vi "carPark.vi"() -> ()   [LabVIEW 2022 SP3]
doc: "This example demonstrates how you can use fuzzy logic to park a vehicle in a specified location."
uses:
  <vilib>/addons/Fuzzy Logic/FL Fuzzy Controller (MISO).vi
  <vilib>/addons/Fuzzy Logic/NI_Fuzzy_Logic_API.lvlib
panel:
  in  "Manual / Fuzzy":bool
  out "Steering Angle":picture
  out "Arrived":bool
  out "Steering Wheel":dbl
  in  "Initial Vehicle Angle":dbl(knob)=-56.0 min=-90.0 max=270.0 step=1.0 scale=-90.0..270.0
  in  "Stop":bool
  out "Grid":cluster{dbl[], dbl[]}[](graph)
  out "Car parking":picture
  # "Garage"
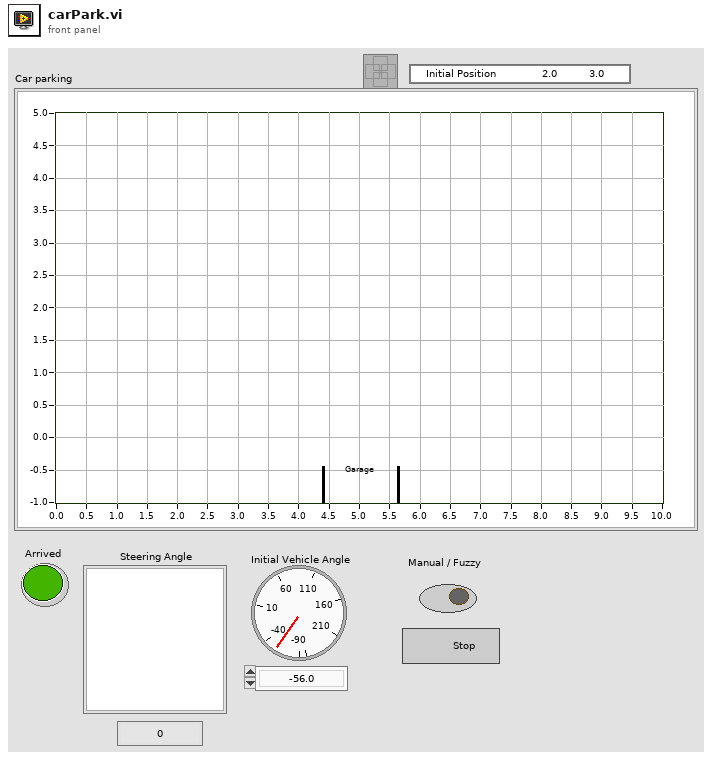
[diagram p1: front panel]
types:
  T1 = typedef "NI_Fuzzy_Logic_API.lvlib/FL System.ctl" = cluster{"input variables":T2[], "output variables":T2[], "rules":T5[], "defuzzification method":T11, "description":string, "user MF interpolating polynomials":T12[]}
  T2 = typedef "NI_Fuzzy_Logic_API.lvlib/FL Variable.ctl" = cluster{"name":string, "range":dbl[], "MFs":T3[]}
  T3 = typedef "NI_Fuzzy_Logic_API.lvlib/FL Membership Function.ctl" = cluster{"name":string, "shape":T4, "points":dbl[], "color":u32, "user-defined shape index":i32}
  T4 = typedef "NI_Fuzzy_Logic_API.lvlib/FL Membership Function Shape.ctl" = u16
  T5 = typedef "NI_Fuzzy_Logic_API.lvlib/FL Rule.ctl" = cluster{"antecedents":T6[], "antecedent connective":T8, "consequents":T9[], "consequent implication":T10, "degree of support":dbl}
  T6 = typedef "NI_Fuzzy_Logic_API.lvlib/FL Antecedent.ctl" = cluster{"Var Index":i32, "MF Index":i32, "Cond":T7}
  T7 = typedef "NI_Fuzzy_Logic_API.lvlib/FL Modifier.ctl" = u16
  T8 = typedef "NI_Fuzzy_Logic_API.lvlib/FL Antecedent Connective.ctl" = u16
  T9 = typedef "NI_Fuzzy_Logic_API.lvlib/FL Consequent.ctl" = cluster{"Var Index":i32, "MF Index":i32, "Cond":T7}
  T10 = typedef "NI_Fuzzy_Logic_API.lvlib/FL Consequent Implication.ctl" = u16
  T11 = typedef "NI_Fuzzy_Logic_API.lvlib/FL Defuzzification.ctl" = u16
  T12 = typedef "NI_Fuzzy_Logic_API.lvlib/FL Interpolating polynomials.ctl" = cluster{"X":dbl[], "Y":dbl[], "Y(x) coeff":dbl[][], "X(y) coeff":dbl[][], "Area(y) coeff":dbl[][], "coa_x(y) coeff":dbl[][]}
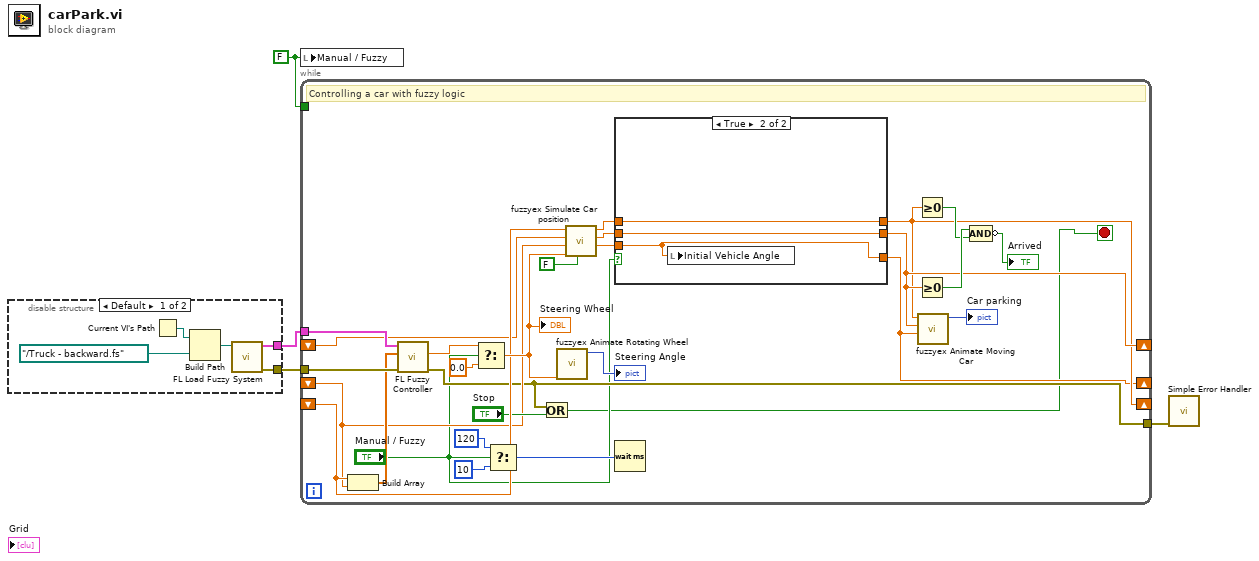
[diagram p0: block diagram]
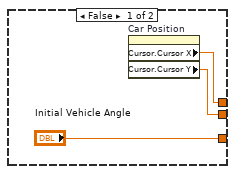
[diagram p3: hidden frame]
diagram:
  w2 = FALSE ("Operation Mode")
  n1 = disable-structure shown="Default" {
    disable-tunnel: [w7 _] -> w4
    disable-tunnel: [w6 _] -> w3
    frame condition #0 (active) {
      n2 = Current VI's Path() -> (path=w5:path)
      n3 = Build Path(base path=w5, name or relative path=path "../Truck - backward.fs") -> (appended path=w9:path)
      n4 = call <vilib>:"FL Load Fuzzy System.vi"("file path"=w9) -> ("error out"=w7:errorcluster, "fuzzy system out"=w6:T1)  [unwired: 1 in, 8 out]
    }
    frame condition #1 {
    }
  }
  n5 = local write "Manual / Fuzzy"(w2) -> ()
  n6 = while {
    shift-left: _ -> [w31]
    shift-right: [w28] -> _
    shift-left: _ -> [w19]
    shift-right: [w27] -> _
    shift-left: _ -> [w18]
    shift-right: [w29] -> _
    tunnel: w2 -> [_]
    tunnel: w3 -> [w30]
    tunnel: w4 -> [w23]
    tunnel: [w15] -> w1
    stop <- w10 stop-if-true
    # "Controlling a car with fuzzy logic"
    n7 = Build Array(w31, w19) -> (w22:dbl[])
    n8 = call-poly <vilib>:"FL Fuzzy Controller.vi"("error in (no error)"=w23, "input values"=w22, "fuzzy system in"=w30) -> ("error out"=w15:errorcluster, "output value"=w12:dbl)  [unwired: 7 out]
    n9 = Select(t=w12, s="Manual / Fuzzy", f=0.0) -> (s? t:f=w33:dbl)
    "Steering Wheel" <- w33
    n10 = Select(t=u32 120, s="Manual / Fuzzy", f=u32 10) -> (s? t:f=w37:u32)
    n11 = Or(x=w15, y="Stop") -> (x .or. y?=w10:bool)
    n12 = call "fuzzyex Animate Rotating Wheel.vi"("Angle (deg)"=w33) -> ("new picture"=→"Steering Angle":picture)  [unwired: 10 out]
    n13 = call "fuzzyex Simulate Car position.vi"("Direction"=FALSE ("f"), "Steering Angle (Phi)"=w33, "Current Vehicle Orientation (Beta)"=w19, "Current Position Y"=w18, "Current Position X"=w31) -> ("New Vehicle Orientation Beta"=w24:dbl, "New position Y"=w25:dbl, "New position X"=w26:dbl)  [unwired: 2 out]
    n14 = case shown="True" "Manual / Fuzzy" {
      tunnel: w25 -> [_ w42]
      tunnel: w26 -> [_ w43]
      tunnel: w24 -> [_ w41]
      tunnel: [w38 w42] -> w29
      tunnel: [w40 w43] -> w28
      tunnel: ["Initial Vehicle Angle" w41] -> w27
      frame False {
        n15 = property on="Car Position" class="XYGraph (strict)"() -> ("Cursor.Cursor X"=w40:dbl, "Cursor.Cursor Y"=w38:dbl)  [unwired: 2 in, 2 out]
      }
      frame True {
        n16 = local write "Initial Vehicle Angle"(w41) -> ()
      }
    }
    n17 = Wait (ms)(milliseconds to wait=w37) -> ()  [unwired: 1 out]
    n18 = Greater Or Equal To 0?(x=w28) -> (x >= 0?=w35:bool)
    n19 = Greater Or Equal To 0?(x=w29) -> (x >= 0?=w36:bool)
    n20 = call "fuzzyex Animate Moving Car.vi"("Car Angle (deg)"=w27, "y position"=w29, "x position"=w28) -> ("new picture"=→"Car parking":picture)  [unwired: 8 out]
    n21 = Compound Arithmetic op=AND(w36, w35) -> (invert →"Arrived":bool)
  }
  n22 = call <vilib>:"Simple Error Handler.vi"("error in (no error)"=w1) -> ()  [unwired: 4 in, 5 out]
